vi "changeTimeScale.vi"(8 "error in (no error)":errorcluster, 10 "timescale":dbl, 11 "AnalysisResultsViewer in":refnum<class "AnalysisResultsViewer.lvclass">) -> (0 "error out":errorcluster, 3 "AnalysisResultsViewer out":refnum<class "AnalysisResultsViewer.lvclass">)   [LabVIEW 2011, in "Views.lvlib" / "Camera.lvlib" / "AnalysisResultsViewer.lvclass"]
uses:
  AnalysisResultsViewer.lvclass
  AnalysisResultsViewer.lvclass/AnalysisResultsViewer.ctl
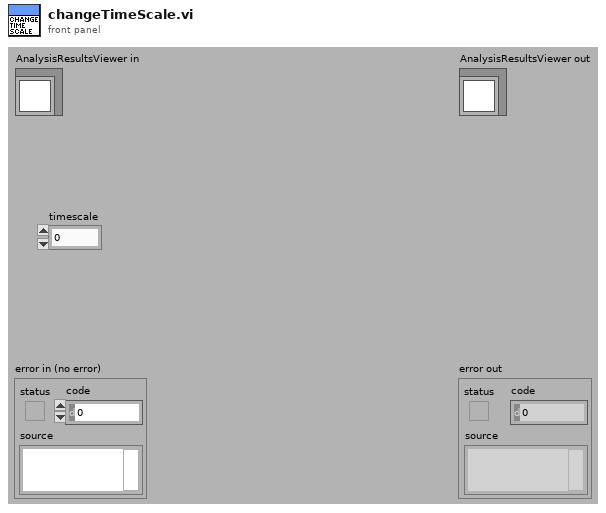
[diagram p1: front panel]
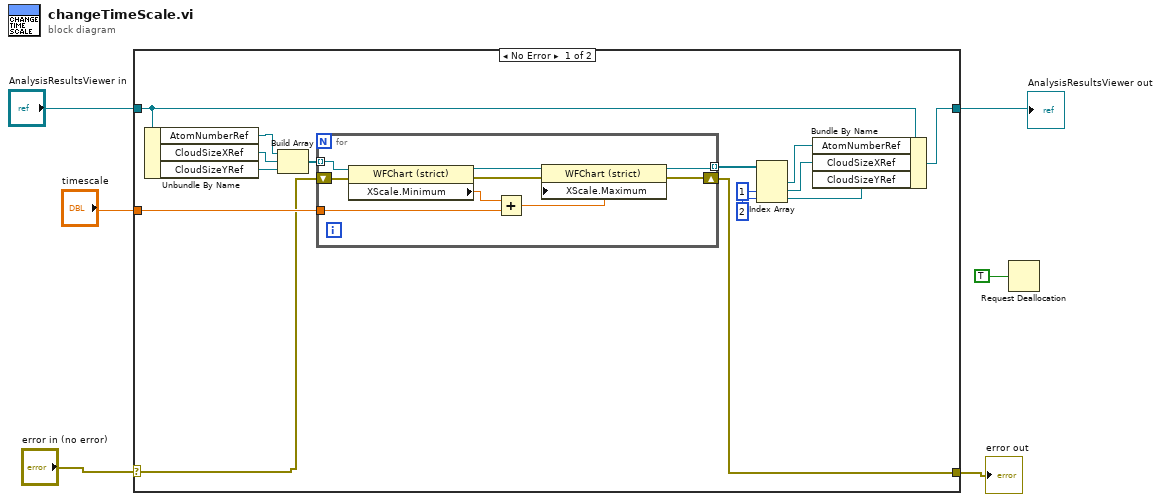
[diagram p0: block diagram]
diagram:
  n1 = case shown="No Error" "error in (no error)" {
    selector: "error in (no error)" -> [w16 w32]
    tunnel: [w15 w32] -> w5
    tunnel: [w7 w31] -> w3
    tunnel: "AnalysisResultsViewer in" -> [w8 w31]
    tunnel: "timescale" -> [w21 _]
    frame No Error {
      n2 = Unbundle By Name(w8) -> ("AtomNumberRef"=w18:refnum<vi>, "CloudSizeXRef"=w19:refnum<vi>, "CloudSizeYRef"=w20:refnum<vi>)
      n3 = Build Array(w18, w19, w20) -> (w17:refnum<vi>[])
      n4 = for {
        tunnel: w21 -> [w27]
        tunnel: w17 -> [w25] mode=indexing
        shift-right: [w22] -> w15
        shift-left: w16 -> [w24]
        tunnel: [w23] -> w14 mode=indexing
        n5 = property class="WFChart (strict)"(reference=w25, error in=w24) -> (reference out=w30:refnum<vi>, error out=w29:errorcluster, "XScale.Minimum"=w28:dbl)
        n6 = Add(x=w28, y=w27) -> (x+y=w26:dbl)
        n7 = property class="WFChart (strict)"(reference=w30, error in=w29, "XScale.Maximum"=w26) -> (reference out=w23:refnum<vi>, error out=w22:errorcluster)
      }
      n8 = Index Array(array=w14, index #2=1, index #3=2) -> (element #1=w9:refnum<vi>, element #2=w10:refnum<vi>, element #3=w11:refnum<vi>)  [unwired: 1 in]
      n9 = Bundle By Name(cluster=w8, "AtomNumberRef"=w9, "CloudSizeXRef"=w10, "CloudSizeYRef"=w11) -> (w7:refnum<class "AnalysisResultsViewer.lvclass">)
    }
    frame Error {
    }
  }
  "error out" <- w5
  "AnalysisResultsViewer out" <- w3
  n10 = Request Deallocation(TRUE ("flag")) -> ()
